vi "Lateral Distance History.vi"(8 "array of clusters":cluster{"Numeric":dbl, "Numeric":dbl}[](array[cluster]), 10 "Trial Index":i32) -> (2 "Lateral Trial History":dbl[][](array[numeric]))   [LabVIEW 2018]
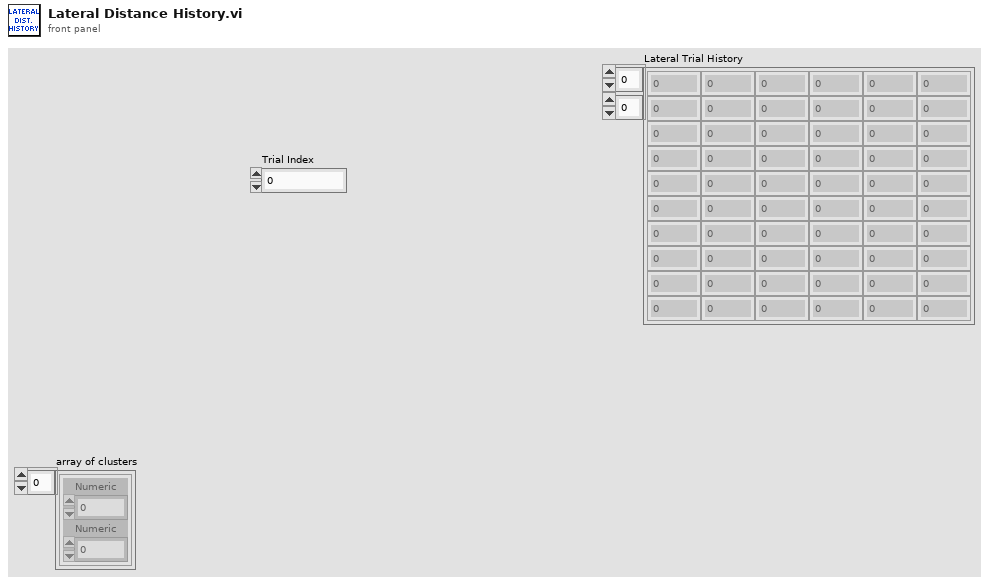
[diagram p1: front panel]
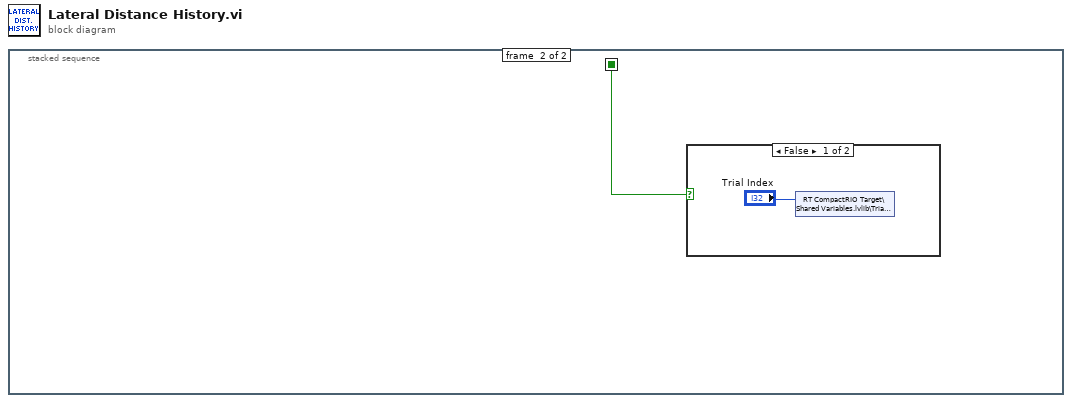
[diagram p0: block diagram]
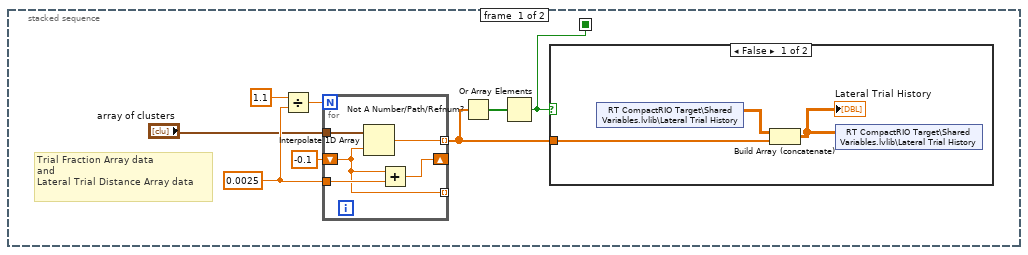
[diagram p2: hidden frame]
diagram:
  n1 = stacked-sequence {
    seq-local: [w1 _] -> [_ w17]
    frame #0 {
      w7 = 0.0025
      # "Trial Fraction Array data\nand\nLateral Trial Distance Array data"
      n2 = Divide(x=1.1, y=w7) -> (x/y=w5:dbl)
      n3 = for {
        N: w5 -> [_]
        tunnel: "array of clusters" -> [w16]
        shift-right: [w15] -> _
        shift-left: -0.1 -> [w12]
        tunnel: [w14] -> w3 mode=indexing
        tunnel: w7 -> [w13]
        tunnel: [w12] -> _ mode=indexing
        n4 = Interpolate 1D Array(1:w12, 2:w16) -> (0:w14:dbl)
        n5 = Add(x=w12, y=w13) -> (x+y=w15:dbl)
      }
      n6 = Not A Number/Path/Refnum?(number/path/refnum=w3) -> (NaN/Path/Refnum?=w2:bool[])
      n7 = Or Array Elements(Boolean array=w2) -> (logical OR=w1:bool)
      n8 = case shown="False" w1 {
        tunnel: w3 -> [w9 _]
        frame False {
          n9 = shared-variable "RT CompactRIO Target\\Shared Variables.lvlib\\Lateral Trial History"() -> (w11:dbl[][])  [unwired: 1 in, 1 out]
          n10 = Build Array (concatenate)(w11, w9) -> (w10:dbl[][])
          "Lateral Trial History" <- w10
          n11 = shared-variable "RT CompactRIO Target\\Shared Variables.lvlib\\Lateral Trial History"(w10) -> ()  [unwired: 1 in, 1 out]
        }
        frame True {
        }
      }
    }
    frame #1 {
      n12 = case shown="False" w17 {
        frame False {
          n13 = shared-variable "RT CompactRIO Target\\Shared Variables.lvlib\\Trial Index"("Trial Index") -> ()  [unwired: 1 in, 1 out]
        }
        frame True {
        }
      }
    }
  }
